vi "Initial MovCor bundler-String.vi"(8 "error in (no error)":errorcluster, 9 "String":T3, 10 "Section name":string, 11 "Refnum in":T2) -> (0 "error out":errorcluster, 3 "Refnum out":T2)   [LabVIEW 2020]
uses:
  <vilib>/Utility/config.llb/Config Data RefNum.ctl
  Typedefs/Ini file interface (String).ctl
  Movement Correction/Typedefs/Control algorithm.ctl
  <vilib>/Utility/config.llb/NI_LVConfig.lvlib
panel:
  out "output 1":T1
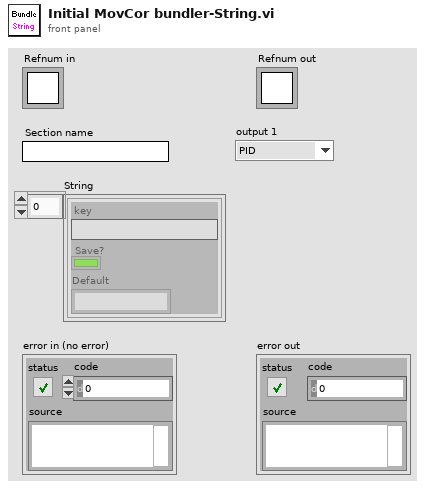
[diagram p1: front panel]
types:
  T1 = typedef "Control algorithm.ctl" = enum16{"PID", "Kalman"}
  T2 = typedef "NI_LVConfig.lvlib/Config Data RefNum.ctl" = refnum<k1>
  T3 = typedef "Ini file interface (String).ctl" = cluster{"key":string, "Save?":bool, "Default":string}[]
  T4 = typedef "Ref DAQ Param.ctl" = cluster{"Full Frame Size":u16, "Ref Field of View":sgl, "Ref Zoom":i8, "Ref_dwellTime":sgl, "Ref X-pixels-per-line(Npxr)":i16, "Ref Y-lines-per-image(Npyr)":i16, "Ref Z-lines-per-image":i16, "Ignore Z lines":i16, "Ref Scan Cycles":i32, "Ref threshold XY":u16, "Ref threshold Z":u16, "Ref average XY":u16, "Ref Average  Z":u16, "Proportional_scale":fxp<+,16,2>, "Integral_scale":fxp<+/-,16,12>, "Proportional_scale Z":fxp<+,16,2>, "Integral_scale Z":fxp<+/-,16,12>, "Diff_threshold":fxp<+,16,2>, "Diff_threshold _z":fxp<+,16,2>, "Sliding Average":bool, "Ref count reset enabled":bool}
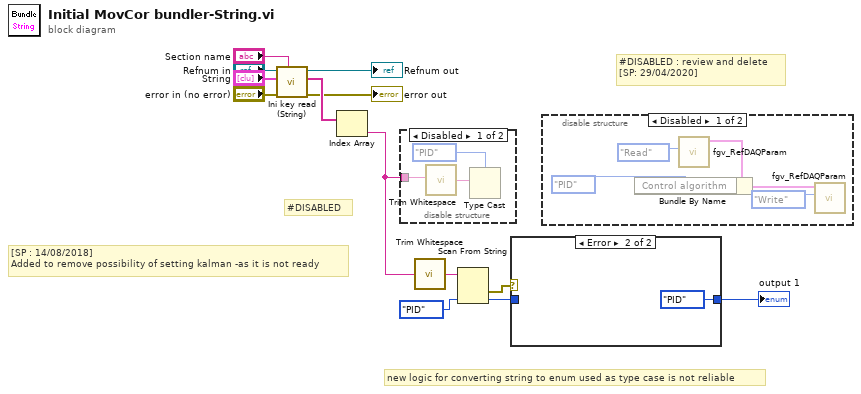
[diagram p0: block diagram]
diagram:
  # "#DISABLED : review and delete\n[SP: 29/04/2020]"
  # "new logic for converting string to enum used as type case is not reliable"
  # "[SP : 14/08/2018]\nAdded to remove possibility of setting kalman -as it is not ready"
  # "#DISABLED"
  n1 = call "Ini key read (String).vi"("Section name"="Section name", "error in (no error)"="error in (no error)", "Keys setup"="String", "Ini file ref in"="Refnum in") -> ("error out"=→"error out":errorcluster, "Value read/used"=w13:string[], "Ini file ref"=→"Refnum out":T2)  [unwired: 5 in]
  n2 = Index Array(array=w13) -> (element=w2:string)  [unwired: 1 in]
  n3 = disable-structure shown="Disabled" {
    disable-tunnel: w2 -> [w16 _]
    frame Disabled {
      n4 = call <vilib>:"Trim Whitespace.vi"("string"=w16) -> ("trimmed string"=w15:string)  [unwired: 1 in]
      n5 = Type Cast(type=Control_algorithm."PID" ("Control algorithm"), x=w15) -> ()  [unwired: 1 out]
    }
    frame Enabled {
    }
  }
  n6 = call <vilib>:"Trim Whitespace.vi"("string"=w2) -> ("trimmed string"=w1:string)  [unwired: 1 in]
  n7 = Scan From String(input string=w1, default 1=Control_algorithm."PID" ("Control algorithm")) -> (error out=w4:errorcluster, output 1=w5:T1)  [unwired: 3 in, 2 out]
  n8 = case shown="Error" w4 {
    tunnel: w5 -> [w17 _]
    tunnel: [w17 Control_algorithm."PID" ("Control algorithm")] -> w3
    frame No Error {
    }
    frame Error {
    }
  }
  "output 1" <- w3
  n9 = disable-structure shown="Disabled" {
    frame Disabled {
      n10 = call "fgv_RefDAQParam.vi"("Function"=enum16{"Initialize", "Write", "Read"}."Read") -> ("RefDAQParam"=w20:T4)  [unwired: 9 in, 1 out]
      n11 = Bundle By Name(cluster=w20, "Control algorithm"=Control_algorithm."PID") -> (w22:T4)
      n12 = call "fgv_RefDAQParam.vi"("Function"=enum16{"Initialize", "Write", "Read"}."Write" ("Status"), "RefDAQParam in"=w22) -> ()  [unwired: 8 in, 2 out]
    }
    frame Enabled {
    }
  }
